vi "ROI group-Obtain ROI indexes in a group.vi"(8 "error in (no error)":errorcluster) -> (0 "error out":errorcluster, 3 "Group's ROIs indexes":i32[](array[numeric]))   [LabVIEW 2013]
uses:
  Typedefs/Get-Set-Clear Control.ctl
  Global variables/gl_Functional Imaging-Global variables.vi
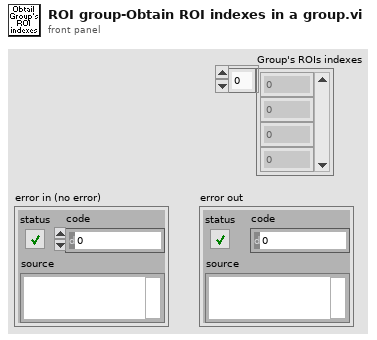
[diagram p1: front panel]
types:
  T1 = typedef "Get-Set-Clear Control.ctl" = enum16{"Get", "Set", "Clear"}
  T2 = typedef "Functional Imging UI Refs.ctl" = cluster{"Menu ref":refnum<k9>, "Image control":refnum<vi>, "VI ref":refnum<vi>, "XGrapher":refnum<vi>, "Smoothing":refnum<vi>, "POI Averaging":refnum<vi>, "Normalize":refnum<vi>, "POI data points in each trial":refnum<vi>, "Channel":refnum<vi>, "Experiment data folder path":refnum<vi>, "[ROI vis]":refnum<vi>, "[Groups] visbl":T3, "Group Name":refnum<vi>, "POI index":refnum<vi>, "Trial No.":refnum<vi>, "Intensity Zoom":refnum<vi>, "Trial Cursor Enabled":refnum<vi>, "Number of Trials (ind 1)":refnum<vi>, "Number of Trials (ind 2)":refnum<vi>, "MiniScans Available":refnum<vi>, "POI Available":refnum<vi>, "Defer graph updates":refnum<vi>, "Waveform selector":refnum<vi>, "#of selected POI":refnum<vi>, "#of selected MiniScans":refnum<vi>, "#of selected groups":refnum<vi>, "Max Z-Projection":refnum<vi>, "Z-Plane Selector":refnum<vi>, "Index of miniscan point to visualise":refnum<vi>, "ROI vis. mode":refnum<vi>, "Total # of points":refnum<vi>, "Index of group clicked on":refnum<vi>, "Pane 1":refnum<vi>, "Pane 2":refnum<vi>, "Pane 3":refnum<vi>, "Pane 4":refnum<vi>, "Pane 5":refnum<vi>, "Pane 6":refnum<vi>, "Deselect all ROI":refnum<vi>, "Deselect all groups":refnum<vi>}
  T3 = typedef "Groups array referecne.ctl" = refnum<vi>
  T4 = typedef "ROI group info cluster.ctl" = cluster{"Group name":string, "# ROI in group":i32, "ROI numbers in group":i32[], "Group region specifier cluster":T5}
  T5 = typedef "ROI Descriptor" = cluster{"Global Rectangle":i32[], "Contours":cluster{"ID":enum32{"External", "Internal"}, "Type":u32, "Coordinates":i32[]}[]}
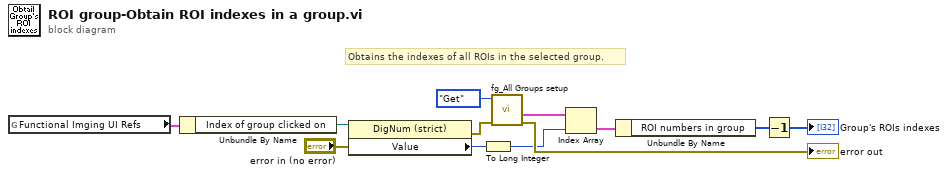
[diagram p0: block diagram]
diagram:
  # "Obtains the indexes of all ROIs in the selected group."
  n1 = global read "gl_Functional Imaging-Global variables.vi" "Functional Imging UI Refs"() -> (w12:T2)
  n2 = Unbundle By Name(w12) -> ("Index of group clicked on"=w11:refnum<vi>)
  n3 = property on="Property Node" class="DigNum (strict)"(reference=w11, error in="error in (no error)") -> (error out=w8:errorcluster, "Value"=w2:i16)  [unwired: 1 out]
  n4 = To Long Integer(number=w2) -> (32bit integer=w1:i32)
  n5 = call "fg_All Groups setup.vi"("error in (no error)"=w8, "Function"=Get-Set-Clear_Control."Get") -> ("error out"=→"error out":errorcluster, "Groups setup out"=w9:T4[])  [unwired: 8 in]
  n6 = Index Array(array=w9, index=w1) -> (element=w7:T4)
  n7 = Unbundle By Name(w7) -> ("ROI numbers in group"=w6:i32[])
  n8 = Decrement(x=w6) -> (x-1=→"Group's ROIs indexes":i32[])
